vi "Fibonacci Numbers.vi"() -> ()   [LabVIEW 2018]
panel:
  out "Numeric":dbl
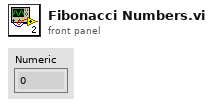
[diagram p1: front panel]
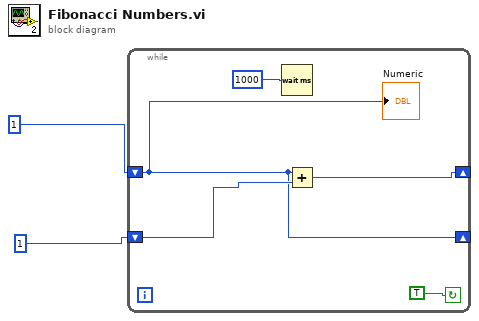
[diagram p0: block diagram]
diagram:
  n1 = while {
    shift-right: [w7] -> _
    shift-left: 1 -> [w4]
    shift-right: [w4] -> _
    shift-left: 1 -> [w5]
    stop <- TRUE continue-if-true
    n2 = Wait (ms)(milliseconds to wait=1000) -> ()  [unwired: 1 out]
    n3 = Add(x=w4, y=w5) -> (x+y=w7:i32)
    "Numeric" <- w4
  }
